vi "checkHandle.vi"(7 "Close all open DDS devices?":bool, 8 "Error In":errorcluster, 10 "DDS Devices":T1(array[cluster])=[{"PB Trigger Line"=21, "Sweeps"=TRUE, "Channel Name"="Evap rf DDS", "Device Description"="Ultracool FPGA 03", "PB trig / Sequence"=TRUE, "Amp Lock"=FALSE, "SetList Display"=[TRUE, FALSE, FALSE], "FPGA Firmware Version"=0.0}, {"PB Trigger Line"=20, "Sweeps"=FALSE, "Channel Name"="Dipole DDS", "Device Description"="Ultracool FPGA 04", "PB trig / Sequence"=TRUE, "Amp Lock"=TRUE, "SetList Display"=[FALSE, TRUE, FALSE], "FPGA Firmware Version"=0.0}, {"PB Trigger Line"=13, "Sweeps"=FALSE, "Channel Name"="2D latt DDS", "Device Description"="Ultracool FPGA 05", "PB trig / Sequence"=TRUE, "Amp Lock"=FALSE, "SetList Display"=[FALSE, TRUE, FALSE], "FPGA Firmware Version"=0.0}, {"PB Trigger Line"=13, "Sweeps"=FALSE, "Channel Name"="Vert latt DDS", "Device Description"="Ultracool FPGA 06", "PB trig / Sequence"=TRUE, "Amp Lock"=FALSE, "SetList Display"=[FALSE, TRUE, FALSE], "FPGA Firmware Version"=0.0}, {"PB Trigger Line"=21, "Sweeps"=TRUE, "Channel Name"="uwave DDS", "Device Description"="Ultracool FPGA 07", "PB trig / Sequence"=TRUE, "Amp Lock"=FALSE, "SetList Display"=[TRUE, TRUE, FALSE], "FPGA Firmware Version"=0.0}], 11 "Previous Device Names and Handles":T2(array[cluster])) -> (0 "error out":errorcluster, 3 "Current Device Names and Handles":T2(array[cluster]))   [LabVIEW 2013, in "DDS9954_v2013.lvlib"]
uses:
  DDS9954_v2013.lvlib
panel:
  # "Freq    Amp   Phase"
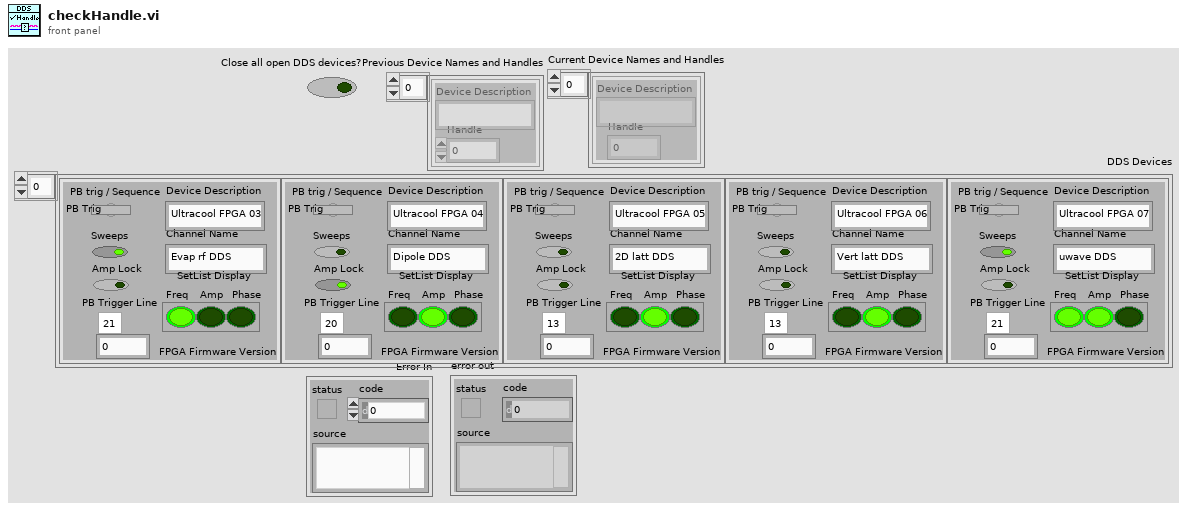
[diagram p1: front panel]
types:
  T1 = cluster{"PB Trigger Line":u16, "Sweeps":bool, "Channel Name":string, "Device Description":string, "PB trig / Sequence":bool, "Amp Lock":bool, "SetList Display":bool[], "FPGA Firmware Version":dbl}[]
  T2 = cluster{"Device Description":string, "Handle":i64}[]
  T3 = cluster{"Device Description":string, "Handle":i64}
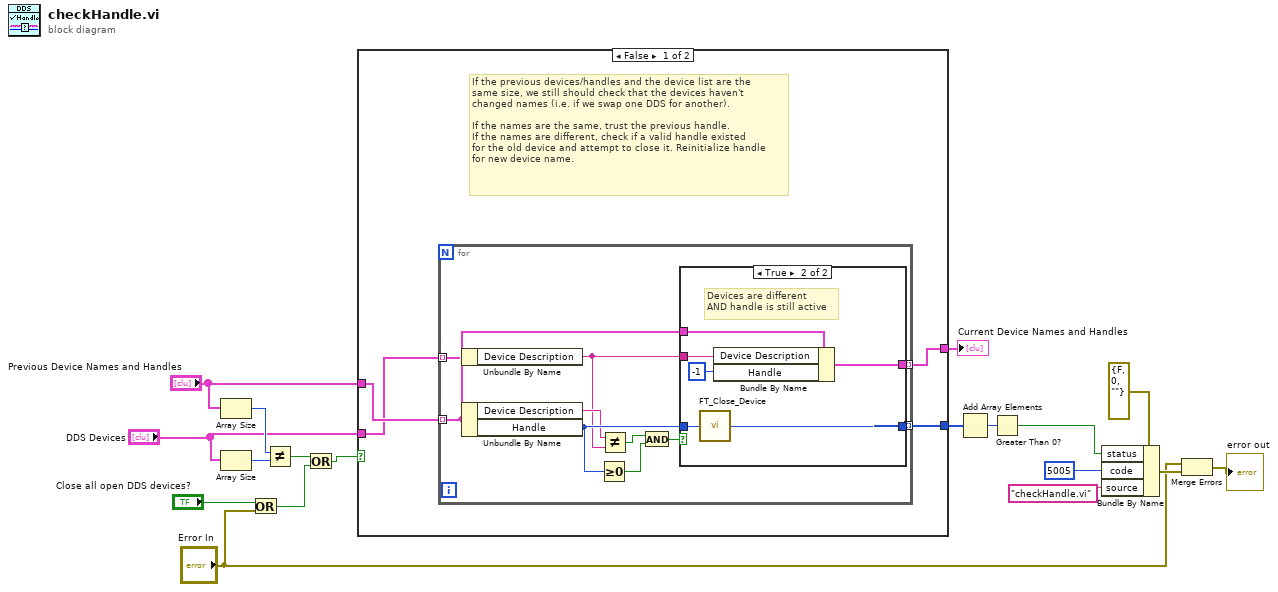
[diagram p0: block diagram]
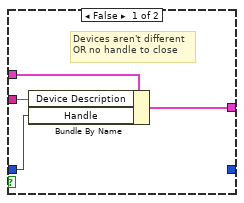
[diagram p2: hidden frame]
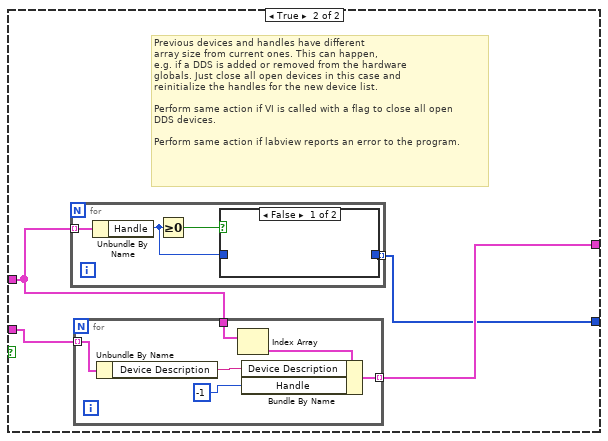
[diagram p3: hidden frame]
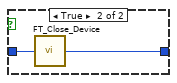
[diagram p4: hidden frame]
diagram:
  n1 = Array Size(array="Previous Device Names and Handles") -> (size(s)=w17:i32)
  n2 = Array Size(array="DDS Devices") -> (size(s)=w18:i32)
  n3 = Or(x="Close all open DDS devices?", y="Error In") -> (x .or. y?=w3:bool)
  n4 = Not Equal?(x=w17, y=w18) -> (x != y?=w6:bool)
  n5 = Or(x=w6, y=w3) -> (x .or. y?=w5:bool)
  n6 = case shown="False" w5 {
    tunnel: "Previous Device Names and Handles" -> [w22 w45]
    tunnel: "DDS Devices" -> [w21 w46]
    tunnel: [w20 w44] -> w15
    tunnel: [w19 w43] -> w14
    frame False {
      # "If the previous devices/handles and the device list are the\nsame size, we still should check that the devices haven't\nchanged names (i.e. if we swap one DDS for another).\n\nIf the names are the same, trust the previous handle.\nIf the names are different, check if a valid handle existed\nfor the old device and attempt to close it. Reinitialize handle\nfor new device name."
      n7 = for {
        tunnel: w22 -> [w27] mode=indexing
        tunnel: w21 -> [w26] mode=indexing
        tunnel: [w24] -> w20 mode=indexing
        tunnel: [w23] -> w19 mode=indexing
        n8 = Unbundle By Name(w26) -> ("Device Description"=w25:string)
        n9 = Unbundle By Name(w27) -> ("Device Description"=w28:string, "Handle"=w32:i64)
        n10 = Greater Or Equal To 0?(x=w32) -> (x >= 0?=w30:bool)
        n11 = Not Equal?(x=w28, y=w25) -> (x != y?=w29:bool)
        n12 = And(x=w29, y=w30) -> (x .and. y?=w31:bool)
        n13 = case shown="True" w31 {
          tunnel: w32 -> [w34 w42]
          tunnel: [_ w41] -> w23
          tunnel: w27 -> [w36 w40]
          tunnel: w25 -> [w35 w38]
          tunnel: [w33 w39] -> w24
          frame False {
            # "Devices aren't different\nOR no handle to close"
            n14 = Bundle By Name(cluster=w36, "Device Description"=w35, "Handle"=w34) -> (w33:T3)
          }
          frame True {
            # "Devices are different\nAND handle is still active"
            n15 = call "FT_Close_Device.vi"("Handle"=w42) -> ("FT_Status"=w41:u32)
            n16 = Bundle By Name(cluster=w40, "Device Description"=w38, "Handle"=i64 -1) -> (w39:T3)
          }
        }
      }
    }
    frame True {
      # "Previous devices and handles have different\narray size from current ones. This can happen,\ne.g. if a DDS is added or removed from the hardware\nglobals. Just close all open devices in this case and\nreinitialize the handles for the new device list.\n\nPerform same action if VI is called with a flag to close all open\nDDS devices.\n\nPerform same action if labview reports an error to the program."
      n17 = for {
        tunnel: w45 -> [w56] mode=indexing
        tunnel: [w53] -> w43 mode=indexing
        n18 = Unbundle By Name(w56) -> ("Handle"=w54:i64)
        n19 = Greater Or Equal To 0?(x=w54) -> (x >= 0?=w55:bool)
        n20 = case shown="False" w55 {
          tunnel: w54 -> [_ w58]
          tunnel: [_ w57] -> w53
          frame False {
          }
          frame True {
            n21 = call "FT_Close_Device.vi"("Handle"=w58) -> ("FT_Status"=w57:u32)
          }
        }
      }
      n22 = for {
        tunnel: w46 -> [w52] mode=indexing
        tunnel: w45 -> [w51]
        tunnel: [w47] -> w44 mode=indexing
        n23 = Unbundle By Name(w52) -> ("Device Description"=w49:string)
        n24 = Index Array(array=w51) -> (element=w50:T3)  [unwired: 1 in]
        n25 = Bundle By Name(cluster=w50, "Device Description"=w49, "Handle"=i64 -1) -> (w47:T3)
      }
    }
  }
  "Current Device Names and Handles" <- w15
  n26 = Add Array Elements(numeric array=w14) -> (sum=w13:u32)
  n27 = Greater Than 0?(x=w13) -> (x > 0?=w8:bool)
  n28 = Bundle By Name(cluster=errorcluster {"status"=FALSE, "code"=0, "source"=""} ("error constant"), "status"=w8, "code"=5005, "source"="checkHandle.vi") -> (w9:errorcluster)
  n29 = Merge Errors("Error In", w9) -> (→"error out":errorcluster)
